vi "Abort.vi"(8 "error in (no error)":errorcluster, 11 "NHRGridSim in":refnum<class "NHRGridSim.lvclass">) -> (0 "error out":errorcluster, 3 "NHRGridSim out":refnum<class "NHRGridSim.lvclass">)   [LabVIEW 2018, in "AcPwrPlugins.lvlib" / "NHRGridSim.lvclass"]
uses:
  NHRGridSim.lvclass
  AcPwrBaseClass/AcPwrBase.lvclass
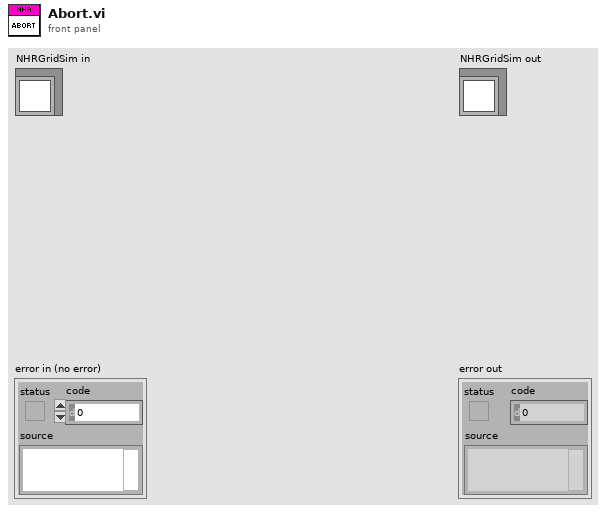
[diagram p1: front panel]
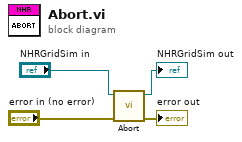
[diagram p0: block diagram]
diagram:
  n1 = call-parent "Abort.vi"("error in (no error)"="error in (no error)", "AcPwrBase in"="NHRGridSim in") -> ("error out"=→"error out":errorcluster, "AcPwrBase out"=→"NHRGridSim out":refnum<class "NHRGridSim.lvclass">)  [unwired: 8 in]
